vi "HAB Climber Global.vi"() -> ()   [LabVIEW 2018]
panel:
  out "HAB Retract":bool
  out "HAB Extend":bool
  out "HAB Retracting limit":bool
  out "HAB Extending limit":bool
  in  "Disable The VI":bool
  in  "Mode":T1(ring)
  in  "State":enum16{"Retracted", "Extended", "Moving", "N/A"}(ring)
  in  "HAB Retract Speed":dbl=-0.3
  in  "HAB Extend Speed":dbl=1.0
  in  "HAB Encoders":dbl
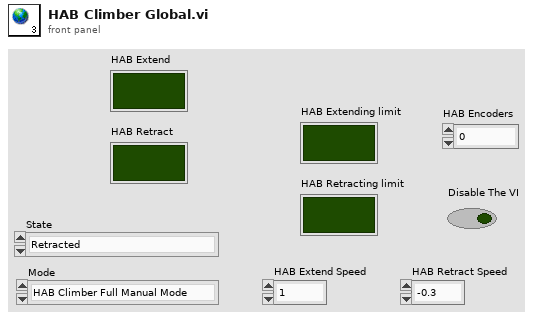
[diagram p1: front panel]
types:
  T1 = enum16{"HAB Climber Full Manual Mode", "HAB Climber Manual Mode", "HAB Climber Automated Mode", "HAB Climber Fully Automated Mode"}
diagram:
